vi "get_size.vi"(8 "error in (no error)":errorcluster, 11 "Box in":refnum<class "Box.lvclass">) -> (0 "error out":errorcluster, 2 "size":refnum<class "SpaceVector.lvclass">, 3 "Box out":refnum<class "Box.lvclass">)   [LabVIEW 2010, in "Box.lvclass"]
uses:
  Box.lvclass
  SpaceVector/SpaceVector/SpaceVector.lvclass
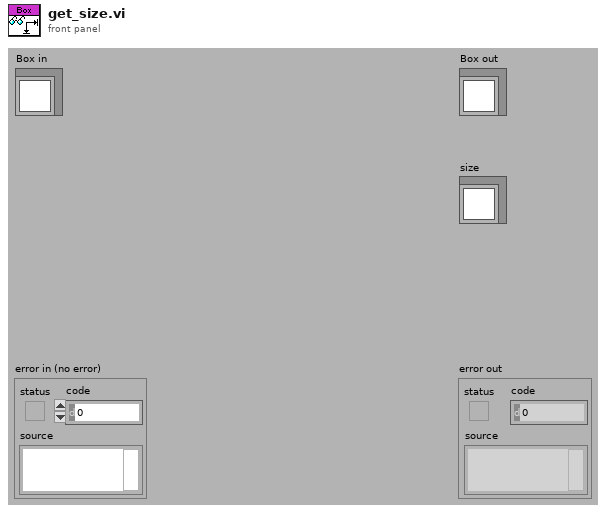
[diagram p1: front panel]
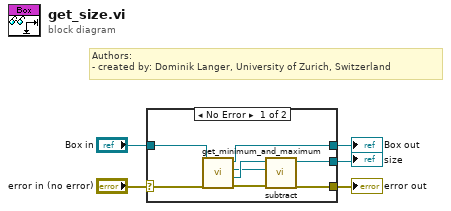
[diagram p0: block diagram]
diagram:
  # "Authors: \n- created by: Dominik Langer, University of Zurich, Switzerland"
  n1 = case shown="No Error" "error in (no error)" {
    selector: "error in (no error)" -> [w10 w15]
    tunnel: [w9 w15] -> w4
    tunnel: [w7 w14] -> w2
    tunnel: "Box in" -> [w8 w14]
    tunnel: [w6 _] -> w1
    frame No Error {
      n2 = call "get_minimum_and_maximum.vi"("error in (no error)"=w10, "Box in"=w8) -> ("error out"=w11:errorcluster, "maximum"=w13:refnum<class "SpaceVector.lvclass">, "minimum"=w12:refnum<class "SpaceVector.lvclass">, "Box out"=w7:refnum<class "Box.lvclass">)  [unwired: 6 in]
      n3 = call "subtract.vi"("error in (no error)"=w11, "subtrahend"=w12, "SpaceVector in"=w13) -> ("error out"=w9:errorcluster, "SpaceVector out"=w6:refnum<class "SpaceVector.lvclass">)  [unwired: 7 in]
    }
    frame Error {
    }
  }
  "error out" <- w4
  "Box out" <- w2
  "size" <- w1
